vi "Communication Handler.vi"(8 "error in":errorcluster, 11 "Message Queues in":T1) -> (0 "error out":errorcluster)   [LabVIEW 2018]
uses:
  support/Message Queue/Message Queue.lvlib
  support/Message Queue/Enqueue Message (Single).vi
  support/Message Queue/Message Cluster.ctl
  support/Message Queue/All Message Queues.ctl
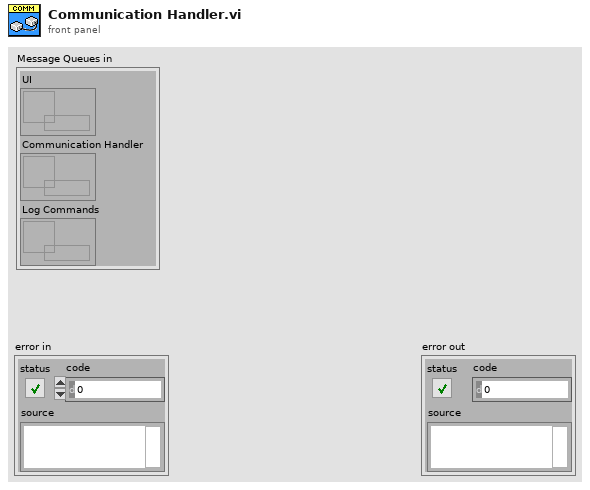
[diagram p1: front panel]
types:
  T1 = typedef "Message Queue.lvlib/All Message Queues.ctl" = cluster{"UI":refnum<queue>, "Communication Handler":refnum<queue>, "Log Commands":refnum<queue>}
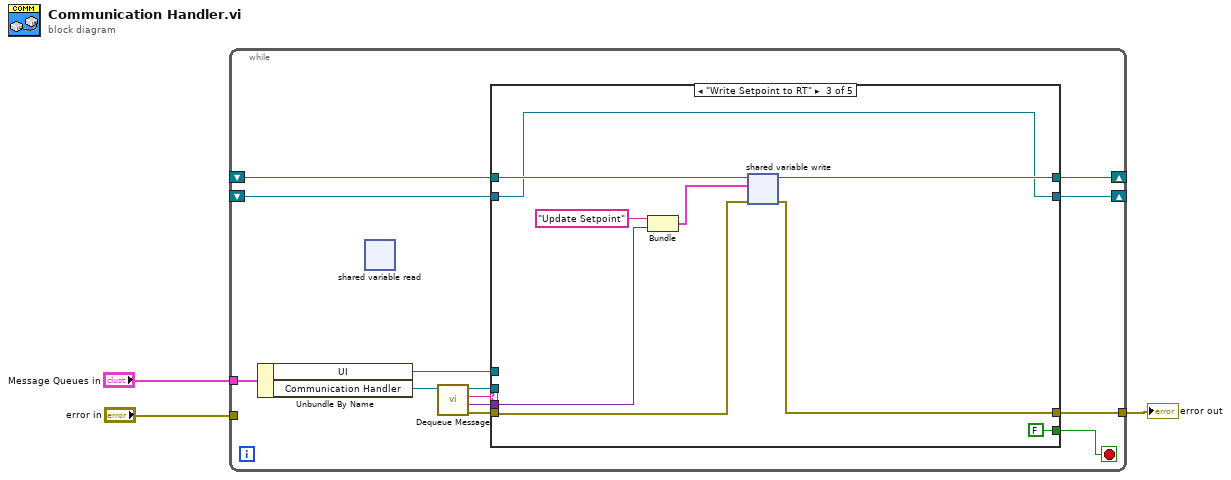
[diagram p0: block diagram]
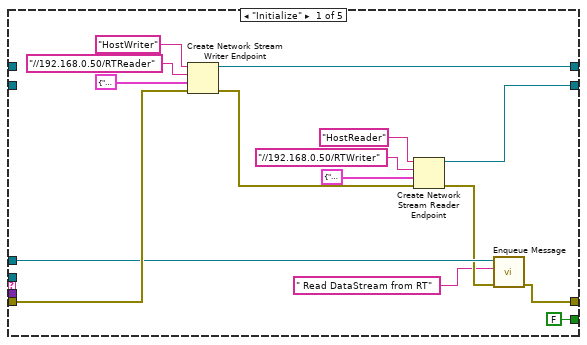
[diagram p2: hidden frame]
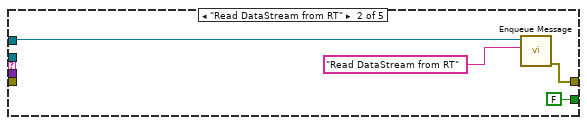
[diagram p3: hidden frame]
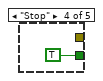
[diagram p4: hidden frame]
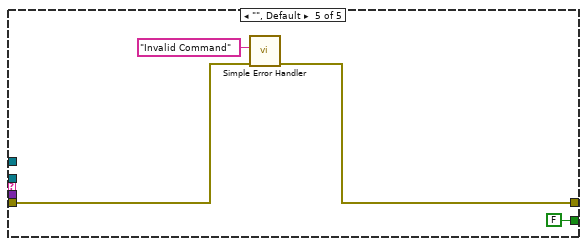
[diagram p5: hidden frame]
diagram:
  n1 = while {
    tunnel: "Message Queues in" -> [w15]
    tunnel: [w10] -> w3
    tunnel: "error in" -> [_]
    shift-right: [w8] -> _
    shift-left: _ -> [w6]
    shift-right: [w7] -> _
    shift-left: _ -> [w5]
    stop <- w9 stop-if-true
    n2 = Unbundle By Name(w15) -> ("UI"=w13:refnum<queue>, "Communication Handler"=w14:refnum<queue>)
    n3 = shared-variable-read() -> ()  [unwired: 4 in, 4 out]
    n4 = call "Dequeue Message.vi"("Message Queue"=w14) -> ("error out"=w11:errorcluster, "Message Data"=w4:variant, "Message"=w16:string, "dup Message Queue"=w12:refnum<queue>)  [unwired: 7 in]
    n5 = case shown="\"Write Setpoint to RT\"" w16 {
      tunnel: w13 -> [w23 w34 _ _ _]
      tunnel: w12 -> [_ _ _ _ _]
      tunnel: w11 -> [w24 _ w39 _ w49]
      tunnel: [w22 w33 w36 _ w47] -> w10
      tunnel: [FALSE FALSE FALSE TRUE FALSE] -> w9
      tunnel: [w18 _ w42 _ _] -> w8
      tunnel: [w17 _ w41 _ _] -> w7
      tunnel: w6 -> [_ _ w43 _ _]
      tunnel: w5 -> [_ _ w41 _ _]
      tunnel: w4 -> [_ _ w38 _ _]
      frame "Initialize" {
        n6 = Create Network Stream Writer Endpoint(8:w24, 9:cluster{string, variant} {"", variant}, 10:"//192.168.0.50/RTReader" ("writer url"), 11:"HostWriter" ("writer name")) -> (0:w25:errorcluster, 3:w18:refnum<k21>)  [unwired: 3 in]
        n7 = Create Network Stream Reader Endpoint(8:w25, 9:cluster{string, variant} {"", variant}, 10:"//192.168.0.50/RTWriter" ("writer url"), 11:"HostReader" ("writer name")) -> (0:w21:errorcluster, 3:w17:refnum<k21>)  [unwired: 3 in]
        n8 = call-poly "Enqueue Message.vi"("error in (no error)"=w21, "Message"=" Read DataStream from RT", "Message Queue"=w23) -> ("error out"=w22:errorcluster)  [unwired: 7 in, 1 out]
      }
      frame "Read DataStream from RT" {
        n9 = call-poly "Enqueue Message.vi"("Message"="Read DataStream from RT", "Message Queue"=w34) -> ("error out"=w33:errorcluster)  [unwired: 8 in, 1 out]
      }
      frame "Write Setpoint to RT" {
        n10 = Bundle("Update Setpoint", "Message Data"=w38) -> (w37:cluster{string, "Message Data":variant})  [unwired: 1 in]
        n11 = shared-variable-write(w43, w39, w37) -> (w42:refnum<k21>, w36:errorcluster)  [unwired: 1 in, 1 out]
      }
      frame "Stop" {
      }
      frame "", Default {
        n12 = call <vilib>:"Simple Error Handler.vi"("error source (\" \")"="Invalid Command" ("error source (\" \")"), "error in (no error)"=w49) -> ("error out"=w47:errorcluster)  [unwired: 3 in, 4 out]
      }
    }
  }
  "error out" <- w3
